vi "ReadAll.vi"(8 "error in (no error)":errorcluster, 11 "NetworkStreamReader in":refnum<class "NetworkStreamReader.lvclass">) -> (0 "error out":errorcluster, 1 "New element?":bool, 2 "elements":variant[](array[variant]), 3 "NetworkStreamReader out":refnum<class "NetworkStreamReader.lvclass">, 4 "Latest time stamp":timestamp)   [LabVIEW 2011, in "NetworkStreamReader.lvclass"]
uses:
  NetworkStreamReader.lvclass
  NetworkStreamReader.lvclass/NetworkStreamReader.ctl
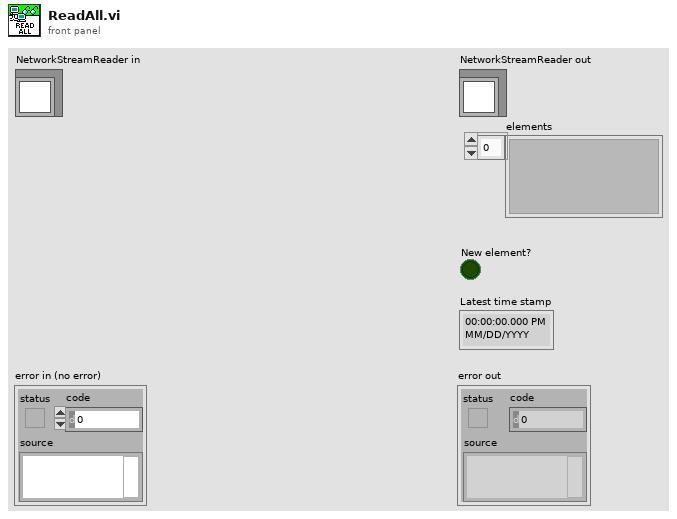
[diagram p1: front panel]
types:
  T1 = typedef "message.ctl" = cluster{"Data":variant, "Time since start (s)":dbl}
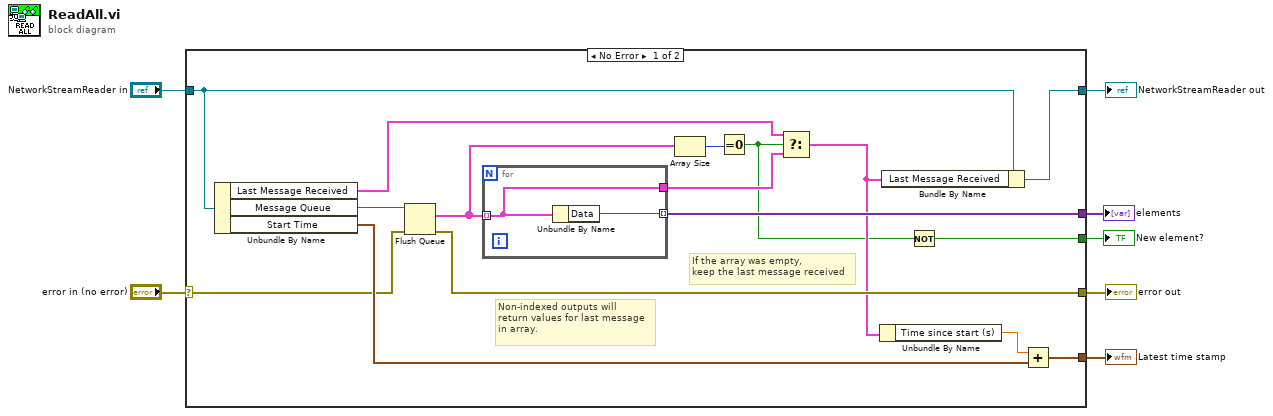
[diagram p0: block diagram]
diagram:
  n1 = case shown="No Error" "error in (no error)" {
    selector: "error in (no error)" -> [w19 w27]
    tunnel: [w17 w27] -> w6
    tunnel: [w22 w26] -> w5
    tunnel: "NetworkStreamReader in" -> [w23 w26]
    tunnel: [w18 _] -> w2
    tunnel: [w20 _] -> w3
    tunnel: [w8 _] -> w1
    frame No Error {
      # "If the array was empty,\nkeep the last message received"
      # "Non-indexed outputs will\nreturn values for last message\nin array."
      n2 = Unbundle By Name(w23) -> ("Last Message Received"=w13:T1, "Message Queue"=w14:refnum<queue>, "Start Time"=w21:timestamp)
      n3 = Flush Queue(queue=w14, error in (no error)=w19) -> (remaining elements=w16:T1[], error out=w17:errorcluster)  [unwired: 1 out]
      n4 = for {
        tunnel: w16 -> [w24] mode=indexing
        tunnel: [w25] -> w18 mode=indexing
        tunnel: [w24] -> w12
        n5 = Unbundle By Name(w24) -> ("Data"=w25:variant)
      }
      n6 = Array Size(array=w16) -> (size(s)=w15:i32)
      n7 = Equal To 0?(x=w15) -> (x = 0?=w9:bool)
      n8 = Select(t=w13, s=w9, f=w12) -> (s? t:f=w11:T1)
      n9 = Unbundle By Name(w11) -> ("Time since start (s)"=w10:dbl)
      n10 = Bundle By Name(cluster=w23, "Last Message Received"=w11) -> (w22:refnum<class "NetworkStreamReader.lvclass">)
      n11 = Not(x=w9) -> (.not. x?=w8:bool)
      n12 = Add(x=w10, y=w21) -> (x+y=w20:timestamp)
    }
    frame Error {
    }
  }
  "error out" <- w6
  "NetworkStreamReader out" <- w5
  "Latest time stamp" <- w3
  "elements" <- w2
  "New element?" <- w1
